vi "Control ROIs Table.vi"(10 "Table":string[][](table), 11 "List ROI in":dbl[][](array[numeric])) -> (3 "ROIs":string[][](table))   [LabVIEW 2023]
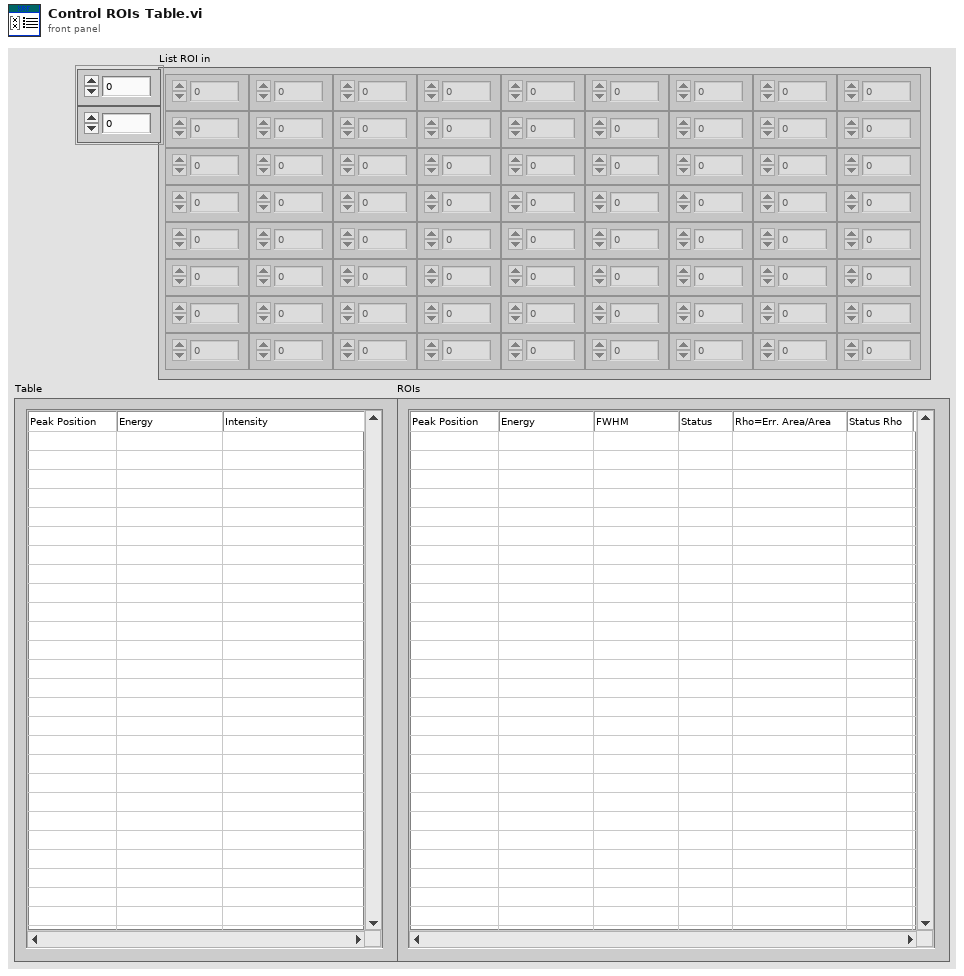
[diagram p1: front panel]
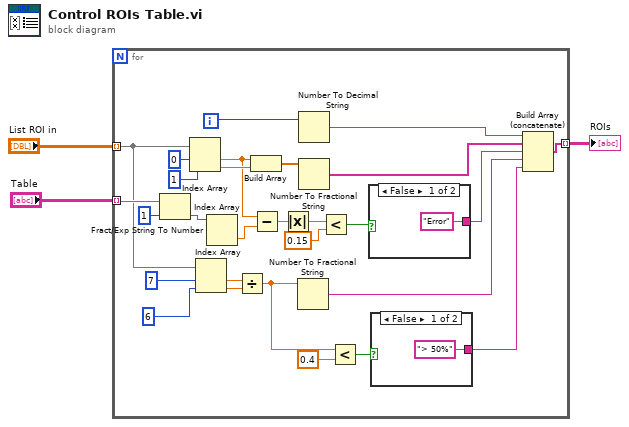
[diagram p0: block diagram]
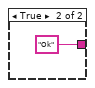
[diagram p2: hidden frame]
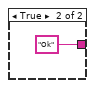
[diagram p3: hidden frame]
diagram:
  n1 = for {
    tunnel: "List ROI in" -> [w13] mode=indexing
    tunnel: [w24] -> w2 mode=indexing
    tunnel: "Table" -> [w23] mode=indexing
    i -> [w27]
    n2 = Index Array(array=w23, index=1) -> (element=w21:string)
    n3 = Index Array(array=w13, index #1=0 ("index"), index #2=1 ("index")) -> (element #1=w20:dbl, element #2=w29:dbl)
    n4 = Index Array(array=w13, index #1=7 ("index"), index #2=6 ("index")) -> (element #1=w9:dbl, element #2=w10:dbl)
    n5 = Fract/Exp String To Number(string=w21) -> (number=w19:dbl)  [unwired: 3 in, 1 out]
    n6 = Divide(x=w9, y=w10) -> (x/y=w6:dbl)
    n7 = Build Array(w20, w29) -> (w28:dbl[])
    n8 = Subtract(x=w20, y=w19) -> (x-y=w18:dbl)
    n9 = Absolute Value(x=w18) -> (abs(x)=w17:dbl)
    n10 = Number To Fractional String(number=w6) -> (F-format string=w8:string)  [unwired: 3 in]
    n11 = Number To Decimal String(number=w27) -> (decimal integer string=w26:string)  [unwired: 1 in]
    n12 = Number To Fractional String(number=w28) -> (F-format string=w25:string[])  [unwired: 3 in]
    n13 = Less?(x=w17, y=0.15) -> (x < y?=w15:bool)
    n14 = Less?(x=w6, y=0.4) -> (x < y?=w7:bool)
    n15 = case shown="False" w15 {
      tunnel: ["Error" "Ok"] -> w14
      frame False {
      }
      frame True {
      }
    }
    n16 = case shown="False" w7 {
      tunnel: ["> 50%" "Ok"] -> w4
      frame False {
      }
      frame True {
      }
    }
    n17 = Build Array (concatenate)(w26, w25, w14, w8, w4) -> (w24:string[])
  }
  "ROIs" <- w2
